vi "_FPGA Set Parameters.vi"(4 "HV Only (F)":bool, 5 "Source Standby (F)":bool, 6 "ExhaustGas (on)":bool=TRUE, 7 "CurGas (on)":bool=TRUE, 8 "error in":errorcluster, 9 "Set Zero (on)":bool=TRUE, 10 "HSID Temp (on)":bool=TRUE, 11 "CurInstrState":T1) -> (0 "error out":errorcluster)   [LabVIEW 2015]
uses:
  Type/_RT Active Ch.ctl
  Type/_RT Instrument State.ctl
  Type/_RT Parameter.ctl
  Type/_RT Expt.ctl
  Type/_Run Mode.ctl
  Type/_RT Mass Range.ctl
  Type/_RT Res Type.ctl
  Type/_FPGA Indicator.ctl
  _RT Global.vi
  <vilib>/Utility/error.llb/Error Cluster From Error Code.vi
  <vilib>/rvi/errors/niLvFpgaAdjustHostInterfaceError.vi
  <vilib>/rvi/interface/nirviReadWriteControl/nirviReadWriteControl.xnode
  Type/FPGA Typedef.ctl
  FPGA Bitfiles/FPGA9607.lvbitx
  NiFpgaLv.dll
panel:
  out "Array":T2[](array[typedef])
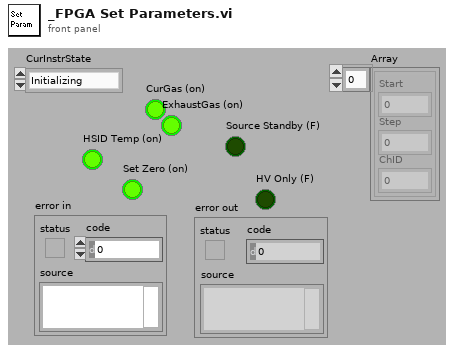
[diagram p1: front panel]
types:
  T1 = typedef "_RT Instrument State.ctl" = enum16{"Initializing", "Mass Spectrometer is Off", "Starting Up", "Turning Power Off", "Going to Standby", "Roughing Pump Ready", "Turning Turbo Off", "Turbo Startup", "Turbopump Ready", "Checking Vacuum", "Going to Ready", "Ready", "Running", "Source Standby", "Lost Communication", "Shutting Down", "Fault", "24V Standby", "Go to 24V Standby", "Turbopump Ready-Waiting"}
  T2 = typedef "_RT Active Ch.ctl" = cluster{"Start":i32, "Step":i32, "ChID":i32}
  T3 = typedef "_RT Expt.ctl" = cluster{"StartT(mS)":i32, "#Cycles":i32, "Scan Type":T4, "PauseT(uS)":i32, "Polarity":u8, "DelayT(mS)":i32, "Active Ch":T2[], "Mass Range":T5[]}
  T4 = typedef "_Run Mode.ctl" = enum16{"MRM (Q1/Q2)", "Q1 Scan", "Q1 SRM", "Q2 Scan", "Q2 SRM", "Product Scan", "Precursor Scan", "Neutral Loss", "Neutral Gain"}
  T5 = typedef "_RT Mass Range.ctl" = cluster{"Steps":i32, "Dwell(uS)":i32, "Resolution Type":T6, "Ramping Ch":T2[]}
  T6 = typedef "_RT Res Type.ctl" = u16
  T7 = typedef "_RT Parameter.ctl" = cluster{"RunMode":i32, "Initial Ch":T2[], "Sync":u8, "Expt":T3[], "EqTime(mS)":i32}
  T8 = typedef "_RT Instrument 2.ctl" = cluster{"Table":T9[], "Instrument":string[]}
  T9 = typedef "_RT Configuration 2.ctl" = cluster{"Name":string, "Ch#":u8, "Min":dbl, "Max":dbl, "Def+":dbl, "Def-":dbl, "Offset":dbl, "Slope":dbl, "Type":u8, "Description":string, "SettleT":dbl}
  T10 = typedef "Semaphore RefNum" = refnum<k1>
  T11 = typedef "_FPGA Indicator.ctl" = enum16{"Done", "Ready", "Count Available", "SendSerial", "LED State"}
  T12 = typedef "FPGA Typedef.ctl" = refnum<k20>
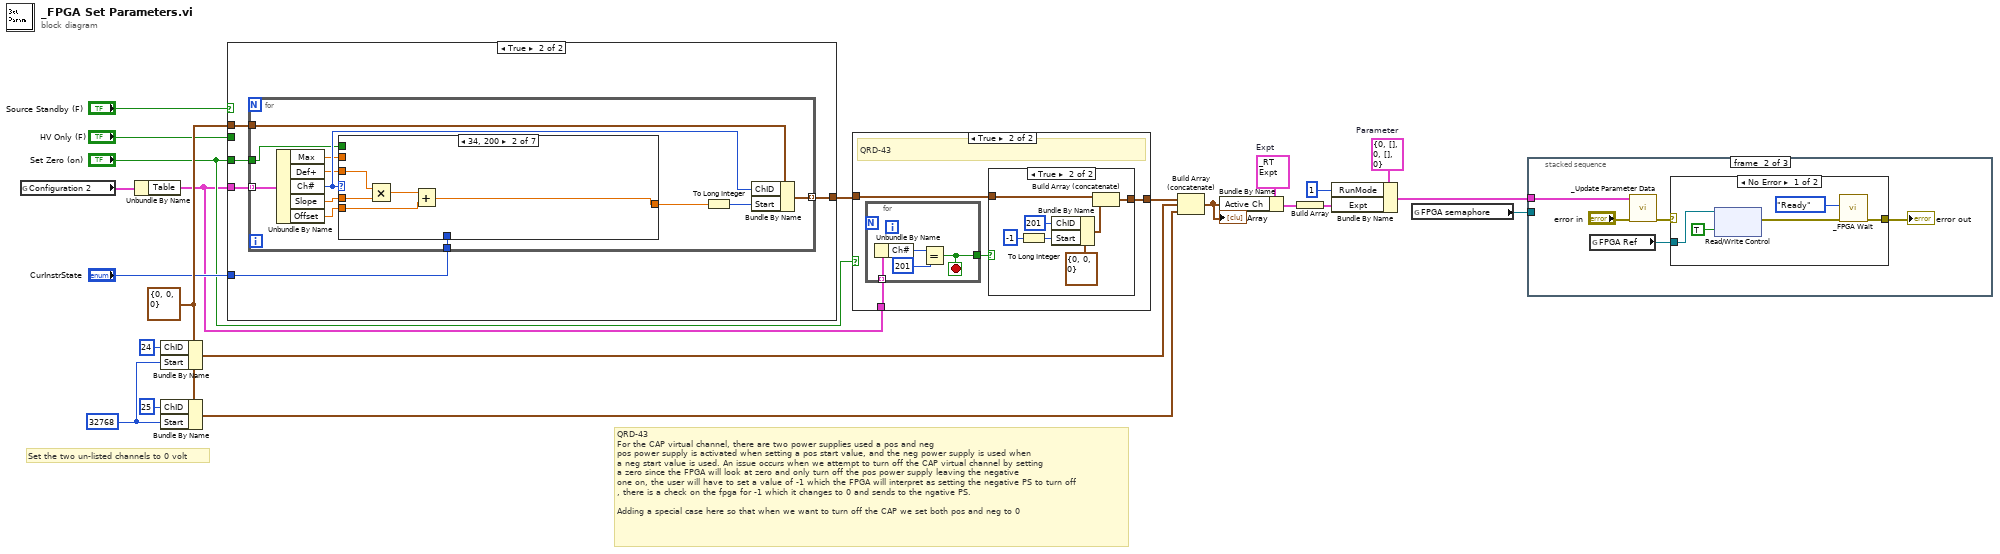
[diagram p0: block diagram]
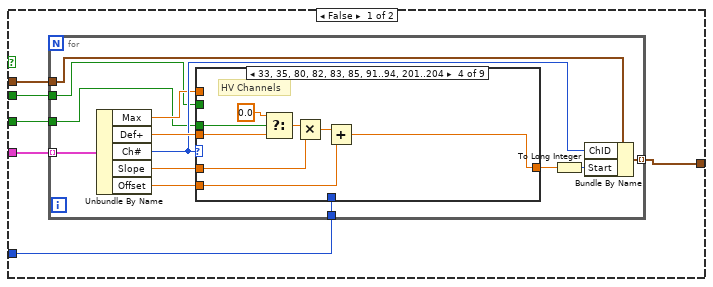
[diagram p4: hidden frame]
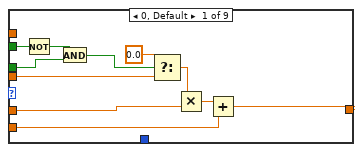
[diagram p5: hidden frame]
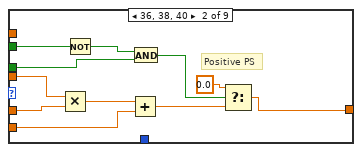
[diagram p6: hidden frame]
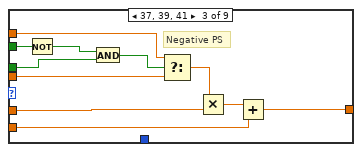
[diagram p7: hidden frame]
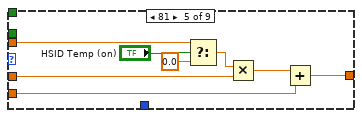
[diagram p8: hidden frame]
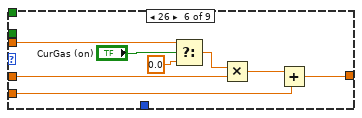
[diagram p9: hidden frame]
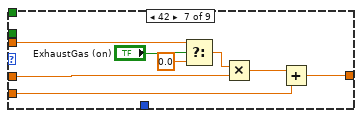
[diagram p10: hidden frame]
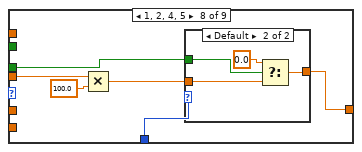
[diagram p11: hidden frame]
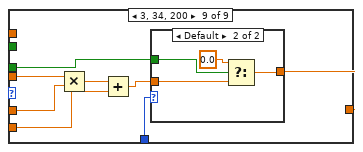
[diagram p13: hidden frame]
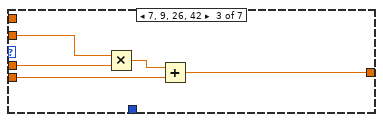
[diagram p16: hidden frame]
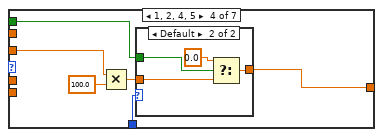
[diagram p17: hidden frame]
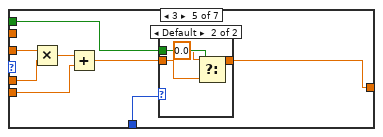
[diagram p19: hidden frame]
diagram:
  w10 = 32768 ("Start")
  w13 = T2 {"Start"=0, "Step"=0, "ChID"=0} ("Active Channel")
  w21 = T3 {"StartT(mS)"=0, "#Cycles"=1, "Scan Type"=enum."MRM (Q1/Q2)", "PauseT(uS)"=0, "Polarity"=0, "DelayT(mS)"=0, "Active Ch"=[], "Mass Range"=[]}  # Expt
  w20 = T7 {"RunMode"=0, "Initial Ch"=[], "Sync"=0, "Expt"=[], "EqTime(mS)"=0}  # Parameter
  # "QRD-43\nFor the CAP virtual channel, there are two power supplies used a pos and neg\npos power supply is activated when setting a pos start value, and the neg power supply is used when\na neg start value is used. An issue occurs when we attempt to turn off the CAP virtual channel by setting\na zero since the FPGA will look at zero and only turn off the pos power supply leaving the negative\none on, the user will have to set a value of -1 which the FPGA will interpret as setting the negative PS to turn off\n, there is a check on the fpga for -1 which it changes to 0 and sends to the ngative PS.\n\nAdding a special case here so that when we want to turn off the CAP we set both pos and neg to 0"
  # "Set the two un-listed channels to 0 volt"
  n1 = global read "_RT Global.vi" "Configuration 2"() -> (w16:T8)
  n2 = Unbundle By Name(w16) -> ("Table"=w1:T9[])
  n3 = Bundle By Name(cluster=w13, "ChID"=24, "Start"=w10) -> (w9:T2)
  n4 = Bundle By Name(cluster=w13, "ChID"=25, "Start"=w10) -> (w8:T2)
  n5 = case shown="True" "Source Standby (F)" {
    tunnel: [w23 w133] -> w4
    tunnel: w1 -> [w24 w134]
    tunnel: w13 -> [w26 w135]
    tunnel: "CurInstrState" -> [w28 w131]
    tunnel: "HV Only (F)" -> [w27 _]
    tunnel: "Set Zero (on)" -> [w25 w132]
    frame False {
      n6 = for {
        tunnel: w24 -> [w41] mode=indexing
        tunnel: [w40] -> w23 mode=indexing
        tunnel: w26 -> [w33]
        tunnel: w28 -> [w31]
        tunnel: w27 -> [w30]
        tunnel: w25 -> [w29]
        n7 = Unbundle By Name(w41) -> ("Max"=w32:dbl, "Def+"=w39:dbl, "Ch#"=w34:u8, "Slope"=w38:dbl, "Offset"=w37:dbl)
        n8 = case shown="33, 35, 80, 82, 83, 85, 91..94, 201..204" w34 {
          tunnel: w39 -> [w44 w55 w65 w78 w85 w92 w100 w111 w125]
          tunnel: w38 -> [w52 w63 w74 w82 w90 w98 w106 _ w121]
          tunnel: w37 -> [w51 w62 w73 w81 w89 w97 w105 _ w120]
          tunnel: [w42 w53 w70 w76 w84 w93 w101 w108 w123] -> w36
          tunnel: w29 -> [w47 w58 w68 w75 _ _ _ w110 w124]
          tunnel: w30 -> [w45 w56 w66 _ _ _ _ _ _]
          tunnel: w32 -> [_ _ w64 _ _ _ _ _ _]
          tunnel: w31 -> [_ _ _ _ _ _ _ w107 w122]
          frame 0, Default {
            n9 = Not(x=w45) -> (.not. x?=w48:bool)
            n10 = And(x=w48, y=w47) -> (x .and. y?=w46:bool)
            n11 = Select(t=0.0 ("f"), s=w46, f=w44) -> (s? t:f=w43:dbl)
            n12 = Multiply(x=w43, y=w52) -> (x*y=w50:dbl)
            n13 = Add(x=w50, y=w51) -> (x+y=w42:dbl)
          }
          frame 36, 38, 40 {
            # "Positive PS"
            n14 = Multiply(x=w55, y=w63) -> (x*y=w61:dbl)
            n15 = Not(x=w56) -> (.not. x?=w59:bool)
            n16 = Add(x=w61, y=w62) -> (x+y=w54:dbl)
            n17 = And(x=w59, y=w58) -> (x .and. y?=w57:bool)
            n18 = Select(t=0.0 ("f"), s=w57, f=w54) -> (s? t:f=w53:dbl)
          }
          frame 37, 39, 41 {
            # "Negative PS"
            n19 = Not(x=w66) -> (.not. x?=w69:bool)
            n20 = And(x=w69, y=w68) -> (x .and. y?=w67:bool)
            n21 = Select(t=w64, s=w67, f=w65) -> (s? t:f=w71:dbl)
            n22 = Multiply(x=w71, y=w74) -> (x*y=w72:dbl)
            n23 = Add(x=w72, y=w73) -> (x+y=w70:dbl)
          }
          frame 33, 35, 80, 82, 83, 85, 91..94, 201..204 {
            # "HV Channels"
            n24 = Select(t=0.0 ("f"), s=w75, f=w78) -> (s? t:f=w77:dbl)
            n25 = Multiply(x=w77, y=w82) -> (x*y=w80:dbl)
            n26 = Add(x=w80, y=w81) -> (x+y=w76:dbl)
          }
          frame 81 {
            n27 = Select(t=w85, s="HSID Temp (on)", f=0.0) -> (s? t:f=w83:dbl)
            n28 = Multiply(x=w83, y=w90) -> (x*y=w88:dbl)
            n29 = Add(x=w88, y=w89) -> (x+y=w84:dbl)
          }
          frame 26 {
            n30 = Select(t=w92, s="CurGas (on)", f=0.0) -> (s? t:f=w91:dbl)
            n31 = Multiply(x=w91, y=w98) -> (x*y=w96:dbl)
            n32 = Add(x=w96, y=w97) -> (x+y=w93:dbl)
          }
          frame 42 {
            n33 = Select(t=w100, s="ExhaustGas (on)", f=0.0) -> (s? t:f=w99:dbl)
            n34 = Multiply(x=w99, y=w106) -> (x*y=w104:dbl)
            n35 = Add(x=w104, y=w105) -> (x+y=w101:dbl)
          }
          frame 1, 2, 4, 5 {
            n36 = Multiply(x=w111, y=100.0) -> (x*y=w109:dbl)
            n37 = case shown="Default" w107 {
              tunnel: w110 -> [_ w117]
              tunnel: w109 -> [w113 w115]
              tunnel: [w113 w114] -> w108
              frame "Source Standby", "Lost Communication" {
              }
              frame Default {
                n38 = Select(t=0.0 ("y"), s=w117, f=w115) -> (s? t:f=w114:dbl)
              }
            }
          }
          frame 3, 34, 200 {
            n39 = Multiply(x=w125, y=w121) -> (x*y=w119:dbl)
            n40 = Add(x=w119, y=w120) -> (x+y=w118:dbl)
            n41 = case shown="Default" w122 {
              tunnel: w124 -> [_ w130]
              tunnel: w118 -> [w126 w128]
              tunnel: [w126 w127] -> w123
              frame "Lost Communication" {
              }
              frame Default {
                n42 = Select(t=0.0 ("y"), s=w130, f=w128) -> (s? t:f=w127:dbl)
              }
            }
          }
        }
        n43 = To Long Integer(number=w36) -> (32bit integer=w35:i32)
        n44 = Bundle By Name(cluster=w33, "ChID"=w34, "Start"=w35) -> (w40:T2)
      }
    }
    frame True {
      n45 = for {
        tunnel: w135 -> [w141]
        tunnel: w134 -> [w140] mode=indexing
        tunnel: [w139] -> w133 mode=indexing
        tunnel: w132 -> [w137]
        tunnel: w131 -> [w136]
        n46 = Unbundle By Name(w140) -> ("Max"=w138:dbl, "Def+"=w143:dbl, "Ch#"=w144:u8, "Slope"=w142:dbl, "Offset"=w147:dbl)
        n47 = case shown="34, 200" w144 {
          tunnel: [w148 w149 w154 w162 w171 w184 0.0 ("Offset")] -> w146
          tunnel: w147 -> [w148 w150 w155 _ w173 w185 _]
          tunnel: w143 -> [_ w152 w157 w161 w176 _ _]
          tunnel: w142 -> [_ w153 w156 _ w175 w186 _]
          tunnel: w138 -> [_ _ _ _ _ w183 _]
          tunnel: w137 -> [_ _ _ w160 w170 _ _]
          tunnel: w136 -> [_ _ _ w159 w177 _ _]
          frame 0, Default {
          }
          frame 34, 200 {
            n48 = Multiply(x=w152, y=w153) -> (x*y=w151:dbl)
            n49 = Add(x=w151, y=w150) -> (x+y=w149:dbl)
          }
          frame 7, 9, 26, 42 {
            n50 = Multiply(x=w157, y=w156) -> (x*y=w158:dbl)
            n51 = Add(x=w158, y=w155) -> (x+y=w154:dbl)
          }
          frame 1, 2, 4, 5 {
            n52 = Multiply(x=w161, y=100.0) -> (x*y=w163:dbl)
            n53 = case shown="Default" w159 {
              tunnel: w160 -> [_ w169]
              tunnel: w163 -> [w165 w167]
              tunnel: [w165 w166] -> w162
              frame "Source Standby", "Lost Communication" {
              }
              frame Default {
                n54 = Select(t=0.0 ("y"), s=w169, f=w167) -> (s? t:f=w166:dbl)
              }
            }
          }
          frame 3 {
            n55 = Multiply(x=w176, y=w175) -> (x*y=w174:dbl)
            n56 = Add(x=w174, y=w173) -> (x+y=w172:dbl)
            n57 = case shown="Default" w177 {
              tunnel: w170 -> [_ w182]
              tunnel: w172 -> [w178 w180]
              tunnel: [w178 w179] -> w171
              frame "Source Standby", "Lost Communication" {
              }
              frame Default {
                n58 = Select(t=0.0 ("y"), s=w182, f=w180) -> (s? t:f=w179:dbl)
              }
            }
          }
          frame 37, 39, 41 {
            # "Negative PS"
            n59 = Multiply(x=w183, y=w186) -> (x*y=w187:dbl)
            n60 = Add(x=w187, y=w185) -> (x+y=w184:dbl)
          }
          frame 36, 38, 40 {
            # "Positive PS"
          }
        }
        n61 = To Long Integer(number=w146) -> (32bit integer=w145:i32)
        n62 = Bundle By Name(cluster=w141, "ChID"=w144, "Start"=w145) -> (w139:T2)
      }
    }
  }
  n63 = case shown="True" "Set Zero (on)" {
    tunnel: w1 -> [_ w192]
    tunnel: w4 -> [w189 w191]
    tunnel: [w189 w190] -> w3
    frame False {
    }
    frame True {
      # "QRD-43"
      n64 = for {
        tunnel: [w203] -> w193
        tunnel: w192 -> [w202] mode=indexing
        stop <- w203 stop-if-true
        n65 = Unbundle By Name(w202) -> ("Ch#"=w205:u8)
        n66 = Equal?(x=w205, y=u8 201) -> (x = y?=w203:bool)
      }
      n67 = case shown="True" w193 {
        tunnel: w191 -> [w194 w199]
        tunnel: [w194 w196] -> w190
        frame False {
        }
        frame True {
          n68 = To Long Integer(number=-1) -> (32bit integer=w201:i32)
          n69 = Bundle By Name(cluster=T2 {"Start"=0, "Step"=0, "ChID"=0} ("Active Channel"), "ChID"=201, "Start"=w201) -> (w198:T2)
          n70 = Build Array (concatenate)(w199, w198) -> (w196:T2[])
        }
      }
    }
  }
  n71 = Build Array (concatenate)(w3, w9, w8) -> (w7:T2[])
  "Array" <- w7
  n72 = Bundle By Name(cluster=w21, "Active Ch"=w7) -> (w18:T3)
  n73 = Build Array(w18) -> (w19:T3[])
  n74 = Bundle By Name(cluster=w20, "RunMode"=1, "Expt"=w19) -> (w22:T7)
  n75 = global read "_RT Global.vi" "FPGA semaphore"() -> (w15:T10)
  n76 = stacked-sequence {
    tunnel: w22 -> [_ w210 _]
    tunnel: w15 -> [w206 _ w218]
    frame #0 {
      n77 = call <vilib>:"Acquire Semaphore.vi"("semaphore"=w206) -> ()  [unwired: 2 in, 5 out]
    }
    frame #1 {
      n78 = global read "_RT Global.vi" "FPGA Ref"() -> (w207:T12)
      n79 = call "_Update Parameter Data.vi"("error in"="error in", "Parameter"=w210) -> ("error out"=w211:errorcluster)  [unwired: 1 in, 4 out]
      n80 = case shown="No Error" w211 {
        selector: w211 -> [_ w217]
        tunnel: w207 -> [w216 _]
        tunnel: [w213 w217] -> w209
        frame No Error {
          n81 = xnode "Read/Write Control"("FPGA VI Reference In"=w216, "Start"=TRUE) -> ("error out"=w212:errorcluster)  [unwired: 1 in, 1 out]
          n82 = call "_FPGA Wait.vi"("error in"=w212, "Indicator"=_FPGA_Indicator."Ready") -> ("error out"=w213:errorcluster)  [unwired: 3 in, 2 out]
        }
        frame Error {
        }
      }
      "error out" <- w209
    }
    frame #2 {
      n83 = call <vilib>:"Release Semaphore.vi"("semaphore"=w218) -> ()  [unwired: 1 in, 6 out]
    }
  }
